vi "Read Channel Info.vi"(8 "error in (no error)":errorcluster, 11 "Readable.lvclass in":refnum<class "Readable.lvclass">) -> (0 "error out":errorcluster, 1 "Channel Units":string[](array[string]), 2 "Channel Names":string[](array[string]), 3 "Readable.lvclass out":refnum<class "Readable.lvclass">, 5 "#Channels":i32)   [LabVIEW 2009, in "Readable.lvclass"]
doc: "(Dynamic) Return information about the readable data channels this object provides, e.g., the name of each data source and its unit."
uses:
  Readable.lvclass
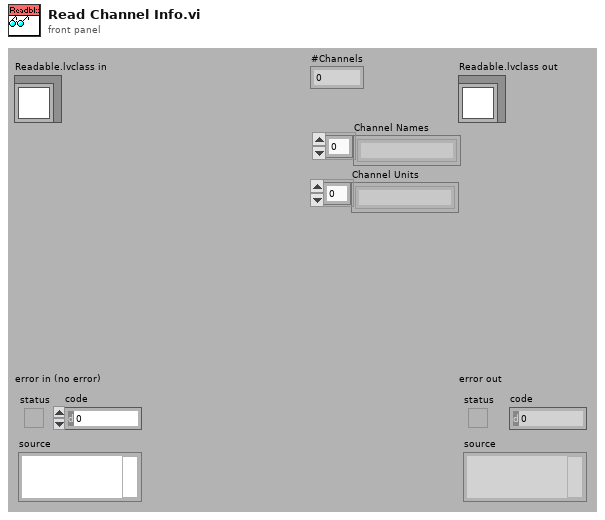
[diagram p1: front panel]
types:
  T1 = typedef "Readable.lvclass/Data Points.ctl" = T2[]
  T2 = typedef "Readable.lvclass/Data Point.ctl" = dbl
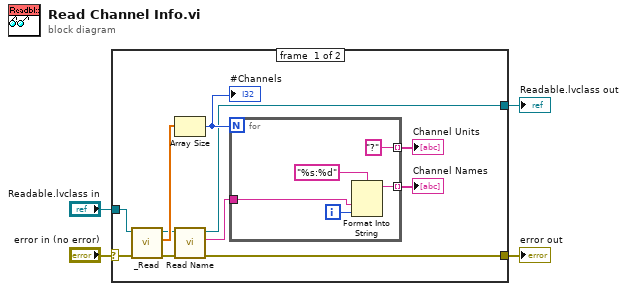
[diagram p0: block diagram]
diagram:
  n1 = case shown="No Error" "error in (no error)" {
    selector: "error in (no error)" -> [w9 w21]
    tunnel: [w7 w21] -> w3
    tunnel: [w5 w22] -> w1
    tunnel: "Readable.lvclass in" -> [w10 w22]
    frame #0 {
      n2 = call-dynamic "_Read.vi"("error in (no error)"=w9, "Readable in"=w10) -> ("error out"=w8:errorcluster, "Data Points"=w11:T1, "Readable out"=w6:refnum<class "Readable.lvclass">)  [unwired: 7 out]
      n3 = Array Size(array=w11) -> (size(s)=w14:i32)
      "#Channels" <- w14
      n4 = call-dynamic "Read Name.vi"("error in (no error)"=w8, "Instrument.lvclass in"=w6) -> ("error out"=w7:errorcluster, "Name"=w15:string, "Instrument.lvclass out"=w5:refnum<class "Readable.lvclass">)  [unwired: 7 out]
      n5 = for {
        N: w14 -> [_]
        tunnel: [w18] -> w13 mode=indexing
        tunnel: w15 -> [w17]
        tunnel: ["?" ("resulting string")] -> w12 mode=indexing
        i -> [w19]
        n6 = Format Into String(format string="%s:%d", w17, w19) -> (resulting string=w18:string)  [unwired: 2 in, 1 out]
      }
      "Channel Names" <- w13
      "Channel Units" <- w12
    }
    frame #1 {
    }
  }
  "error out" <- w3
  "Readable.lvclass out" <- w1
